vi "Remove Settings.vi"(8 "error in (no error)":errorcluster, 10 "setting ID":string, 11 "Configuration Session in":refnum<class "Configuration Session.lvclass">) -> (0 "error out":errorcluster, 3 "Configuration Session out":refnum<class "Configuration Session.lvclass">, 4 "exists?":bool)   [LabVIEW 2017, in "DSF Core.lvlib" / "Configuration Session.lvclass"]
doc: "Removes a section from the configuration data identified by <B>dsf refnum</B>."
uses:
  Configuration Session.lvclass
  Configuration Session.lvclass/Configuration Session.ctl
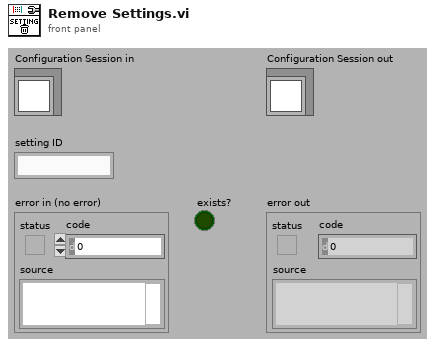
[diagram p1: front panel]
types:
  T1 = typedef "DSF Core.lvlib/Configuration Session.lvclass/DSF Config Data Ref.ctl" = refnum<data-value>
  T2 = typedef "DSF Core.lvlib/Configuration Session.lvclass/DSF Config Data.ctl" = cluster{"dsf configuration":T3, "path":path, "dirty":bool}
  T3 = typedef "DSF Core.lvlib/Configuration Session.lvclass/Internal DSF Configuration.ctl" = cluster{"dsfversion":T4, "version":T4, "plugins":T5[], "groups":T8[], "transfers":T10[], "channels":T12[], "settings":T14[]}
  T4 = typedef "DSF Core.lvlib/DSF Version Info.ctl" = cluster{"major":u32, "minor":u32, "fix":u32, "build":string}
  T5 = typedef "DSF Core.lvlib/Configuration Session.lvclass/Internal DSF Plugin with ID.ctl" = cluster{"id":string, "values":T6}
  T6 = typedef "DSF Core.lvlib/Configuration Session.lvclass/Internal DSF Plugin Info.ctl" = cluster{"type":string, "timing":T7, "group ids":string[], "settings id":string, "thread count":i32}
  T7 = typedef "DSF Core.lvlib/DSF Timing Info.ctl" = cluster{"priority":u64, "decimation":u64, "offset":u64}
  T8 = typedef "DSF Core.lvlib/Configuration Session.lvclass/Internal DSF Group with ID.ctl" = cluster{"id":string, "values":T9}
  T9 = typedef "DSF Core.lvlib/Configuration Session.lvclass/Internal DSF Group Info.ctl" = cluster{"direction":i32, "timing":T7, "transfer ids":string[], "settings id":string}
  T10 = typedef "DSF Core.lvlib/Configuration Session.lvclass/Internal DSF Transfer with ID.ctl" = cluster{"id":string, "values":T11}
  T11 = typedef "DSF Core.lvlib/Configuration Session.lvclass/Internal DSF Transfer Info.ctl" = cluster{"byte order":i32, "channel ids":string[], "settings id":string}
  T12 = typedef "DSF Core.lvlib/Configuration Session.lvclass/Internal DSF Channel with ID.ctl" = cluster{"id":string, "values":T13}
  T13 = typedef "DSF Core.lvlib/Configuration Session.lvclass/Internal DSF Channel Info.ctl" = cluster{"count":u64, "buffer offset":u64, "data type":i32, "settings id":string}
  T14 = typedef "DSF Core.lvlib/Configuration Session.lvclass/Internal DSF Settings with ID.ctl" = cluster{"id":string, "values":T15}
  T15 = typedef "DSF Core.lvlib/Configuration Session.lvclass/Internal DSF Settings Info.ctl" = cluster{"key":string, "value":string}[]
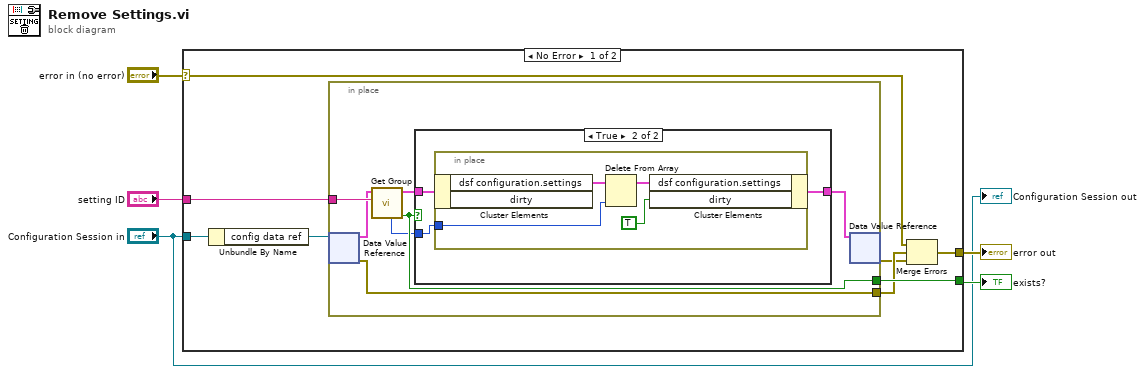
[diagram p0: block diagram]
diagram:
  n1 = case shown="No Error" "error in (no error)" {
    selector: "error in (no error)" -> [w8 w29]
    tunnel: [w11 w29] -> w2
    tunnel: "Configuration Session in" -> [w7 _]
    tunnel: "setting ID" -> [w13 _]
    tunnel: [w12 _] -> w3
    frame No Error {
      n2 = Unbundle By Name(w7) -> ("config data ref"=w6:T1)
      n3 = in-place {
        in-place-border: w13 -> [w20]
        in-place-border: [w19] -> w12
        in-place-border: [w14] -> w10
        n4 = in-place-dvr #1(w6) -> (w16:T2, w14:errorcluster)
        n5 = call "Get Group.vi"("id"=w20, "DSF Configuration in"=w16) -> ("exists?"=w19:bool, "DSF Configuration out"=w18:T2, "index"=w17:i32)  [unwired: 6 in, 1 out]
        n6 = case shown="True" w19 {
          tunnel: [w21 w24] -> w15
          tunnel: w17 -> [_ w23]
          tunnel: w18 -> [w21 w22]
          frame False {
          }
          frame True {
            n7 = in-place {
              in-place-border: w23 -> [w28]
              n8 = in-place-cluster #2(w22) -> ("dsf configuration.settings"=w27:T14[])  [unwired: 1 out]
              n9 = Delete From Array(array=w27, index=w28) -> (array with subset deleted=w26:T14[])  [unwired: 1 in, 1 out]
              n10 = in-place-cluster #2("dsf configuration.settings"=w26, "dirty"=TRUE) -> (w24:T2)
            }
          }
        }
        n11 = in-place-dvr #1(w15) -> (w9:errorcluster)  [unwired: 1 out]
      }
      n12 = Merge Errors(w8, w10, w9) -> (w11:errorcluster)
    }
    frame Error {
    }
  }
  "error out" <- w2
  "exists?" <- w3
  "Configuration Session out" <- "Configuration Session in"
